vi "Natural String Merge Sort.vi"(11 "Array in":cluster{"Key":string, "Value":variant}[](array[cluster])) -> (3 "Array out":cluster{"Key":string, "Value":variant}[](array[cluster]))   [LabVIEW 2020, in "UI Common.lvlib"]
uses:
  UI Common.lvlib
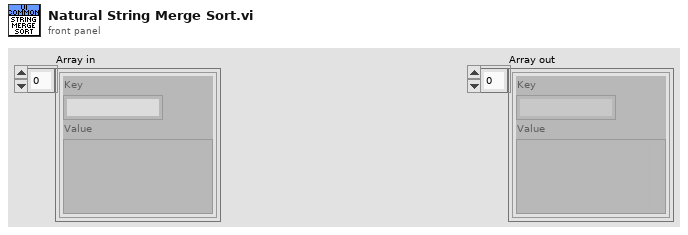
[diagram p1: front panel]
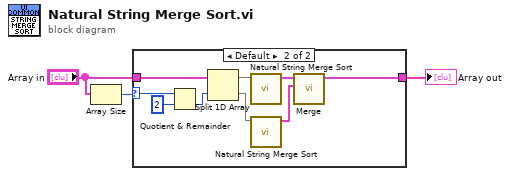
[diagram p0: block diagram]
diagram:
  n1 = Array Size(array="Array in") -> (size(s)=w3:i32)
  n2 = case shown="Default" w3 {
    selector: w3 -> [_ w10]
    tunnel: "Array in" -> [w4 w8]
    tunnel: [w4 w11] -> w1
    frame 0, 1 {
    }
    frame Default {
      n3 = Quotient & Remainder(x=w10, y=2) -> (floor(x/y)=w7:i32)  [unwired: 1 out]
      n4 = Split 1D Array(array=w8, index=w7) -> (first subarray=w6:cluster{"Key":string, "Value":variant}[], second subarray=w5:cluster{"Key":string, "Value":variant}[])
      n5 = call "Natural String Merge Sort.vi"("Array in"=w6) -> ("Array out"=w13:cluster{"Key":string, "Value":variant}[])  [unwired: 10 in]
      n6 = call "Natural String Merge Sort.vi"("Array in"=w5) -> ("Array out"=w12:cluster{"Key":string, "Value":variant}[])  [unwired: 10 in]
      n7 = call "Merge.vi"("Array 2"=w12, "Array 1"=w13) -> ("Array"=w11:cluster{"Key":string, "Value":variant}[])  [unwired: 9 in]
    }
  }
  "Array out" <- w1
